vi "Set Error Tunnel Use Default If not Connected.vi"(8 "error in (no error)":errorcluster, 10 "Use Default if Unwired":bool=TRUE, 11 "CSM-Helper in":refnum<class "CSM-Helper.lvclass">) -> (0 "error out":errorcluster, 3 "CSM-Helper out":refnum<class "CSM-Helper.lvclass">)   [LabVIEW 2017, in "CSM-Helper.lvclass"]
doc: "### Set Error Tunnel Use Default If not Connected.vi\n\n-- <b>Controls</b> --\n- <b>Use Default if not wired</b>:\n- <b>CSM-Helper in</b>: CSMHelper input\n\n-- <b>Indicators</b> --\n- <b>CSM-Helper out</b>: CSMHelper output"
uses:
  CSM-Helper.lvclass
  CSM-Helper.lvclass/CSM-Helper.ctl
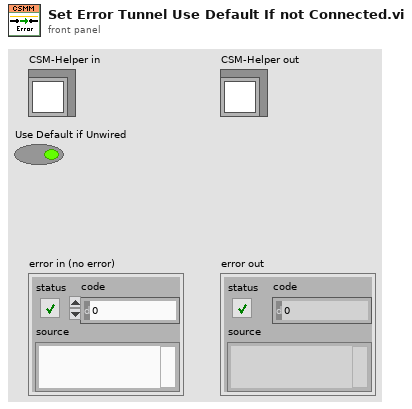
[diagram p1: front panel]
types:
  T1 = typedef "CSM-Helper.lvclass/_csmhelper_Back_Tunnels_Refs.ctl" = cluster{"Registration":refnum<vi>, "InternalData":refnum<vi>, "Resp":refnum<vi>, "Remaining State":refnum<vi>, "Error":refnum<vi>}
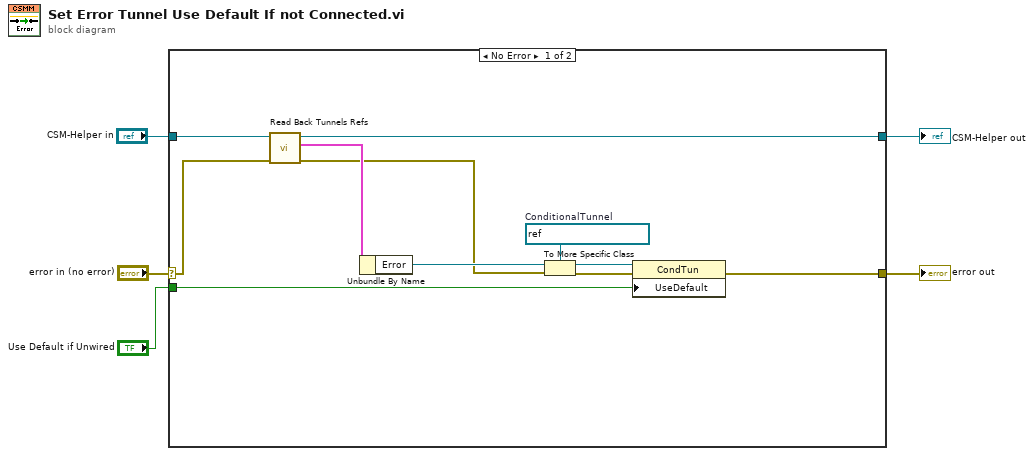
[diagram p0: block diagram]
diagram:
  n1 = case shown="No Error" "error in (no error)" {
    selector: "error in (no error)" -> [w13 w18]
    tunnel: "CSM-Helper in" -> [w15 w17]
    tunnel: [w14 w17] -> w4
    tunnel: [w12 w18] -> w2
    tunnel: "Use Default if Unwired" -> [w6 _]
    frame No Error {
      w9 = refnum<vi> refnum  # ConditionalTunnel
      n2 = call "Read Back Tunnels Refs.vi"("error in (no error)"=w13, "CSM-Helper in"=w15) -> ("error out"=w8:errorcluster, "Back Tunnels"=w16:T1, "CSM-Helper out"=w14:refnum<class "CSM-Helper.lvclass">)  [unwired: 7 in]
      n3 = Unbundle By Name(w16) -> ("Error"=w11:refnum<vi>)
      n4 = To More Specific Class(target class=w9, reference=w11, error in=w8) -> (specific class reference=w10:refnum<vi>, error out=w7:errorcluster)
      n5 = property class="CondTun"(reference=w10, error in=w7, "UseDefault"=w6) -> (error out=w12:errorcluster)  [unwired: 1 out]
    }
    frame Error {
    }
  }
  "CSM-Helper out" <- w4
  "error out" <- w2
